vi "Get Resource ID.vi"(4 "AnalogIn in":refnum<class "AI.lvclass">) -> (7 "Resource ID":string)   [LabVIEW 2020, in "CTI.lvlib" / "AI.lvclass"]
uses:
  AI.lvclass
  AI.lvclass/AI.ctl
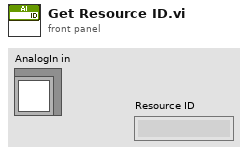
[diagram p1: front panel]
types:
  T1 = typedef "CTI.lvlib/ADC Number.ctl" = i8
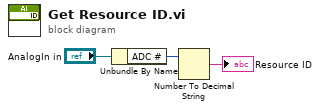
[diagram p0: block diagram]
diagram:
  n1 = Unbundle By Name("AnalogIn in") -> ("ADC #"=w2:T1)
  n2 = Number To Decimal String(number=w2) -> (decimal integer string=→"Resource ID":string)  [unwired: 1 in]
